vi "Get API Version.vi"(8 "error in (no error)":errorcluster, 11 "Hardware Ref in":T1 format="%.0x") -> (0 "error out":errorcluster, 2 "API version":u32, 3 "Hardware Ref out":T1 format="%.0x", 4 "Found?":bool)   [LabVIEW 2020, in "Routing and Faulting Hardware API.lvlib"]
doc: "Gets the version of the Routing and Faulting Hardware API for the given instance of a Routing and Faulting Hardware Custom Device."
uses:
  Routing and Faulting Hardware API.lvlib
  <vilib>/NI VeriStand/Custom Device API/Custom Device Item Ref.ctl
  Routing and Faulting Hardware API Constants.vi
  <vilib>/NI VeriStand/Custom Device API/Get Item Property (U32).vi
  <vilib>/NI VeriStand/Custom Device API/Custom Device API.lvlib
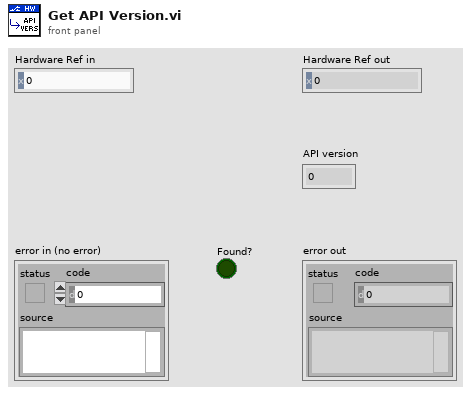
[diagram p1: front panel]
types:
  T1 = typedef "Custom Device API.lvlib/Custom Device Item Ref.ctl" = u64
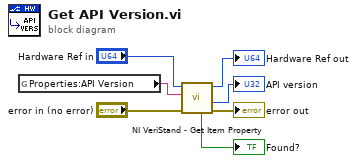
[diagram p0: block diagram]
diagram:
  n1 = global read "Routing and Faulting Hardware API Constants.vi" "Properties:API Version"() -> (w2:string)
  n2 = call-poly <vilib>:"NI VeriStand - Get Item Property.vi"("error in (no error)"="error in (no error)", "Property Name"=w2, "Item Ref in"="Hardware Ref in") -> ("error out"=→"error out":errorcluster, "Value"=→"API version":u32, "Item Ref out"=→"Hardware Ref out":T1, "Found?"=→"Found?":bool)  [unwired: 5 in]
